vi "GetMemory_byPtr.vi"(4 "Data Type":variant, 5 "error in (no error)":errorcluster, 7 "Data Size(1)":i32=1, 8 "Pointer":i32) -> (0 "error out":errorcluster, 2 "data":string, 3 "Duplicate Pointer":i32)   [LabVIEW 2011]
doc: "This VI returns a specified block of memory from a memory pointer. Data is returned as a flattened data string, exactly the way it was in memory. If the <B>Type</B> input is wired, then the VI returns a memory block for#<B>Data Size</B> elements of that type. Otherwise, <B>Data Size</B> refers to the number of bytes to return."
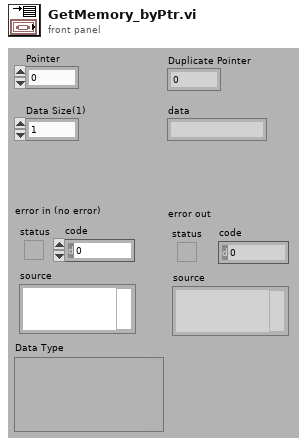
[diagram p1: front panel]
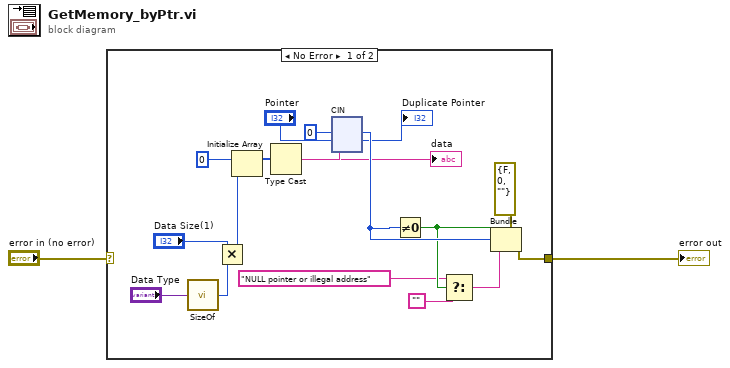
[diagram p0: block diagram]
diagram:
  n1 = case shown="No Error" "error in (no error)" {
    selector: "error in (no error)" -> [_ w21]
    tunnel: [w19 w21] -> w1
    frame No Error {
      n2 = call "SizeOf.vi"("Data"="Data Type") -> ("Size"=w6:i32)
      n3 = Multiply(x="Data Size(1)", y=w6) -> (x*y=w5:i32)
      n4 = Initialize Array(u8 0, w5) -> (w14:u8[])
      n5 = Type Cast(x=w14) -> (*(type *) &x=w13:string)  [unwired: 1 out]
      n6 = cin(0, "Pointer", w13) -> (w16:i32, →"Duplicate Pointer":i32, →"data":string)
      n7 = Not Equal To 0?(x=w16) -> (x != 0?=w12:bool)
      n8 = Select(t="NULL pointer or illegal address", s=w12, f="") -> (s? t:f=w9:string)
      n9 = Bundle(cluster=errorcluster {"status"=FALSE, "code"=0, "source"=""} ("error in (no error)"), "status"=w12, "code"=w16, "source"=w9) -> (w19:errorcluster)
    }
    frame Error {
    }
  }
  "error out" <- w1
